vi "ALTS-2015 Delete User Account v1.0.vi"(8 "error in (no error)":errorcluster, 11 "Last User":string) -> (0 "error out":errorcluster)   [LabVIEW 2013]
panel:
  in  "Case Constant\n(See Context Help)":bool
  out "Time":string
  in  "User Name":i32(ring) items=["Administrator", "Senthil"]
  in  "Cancel":bool
  in  "Delete":bool
  # "Delete User Account"
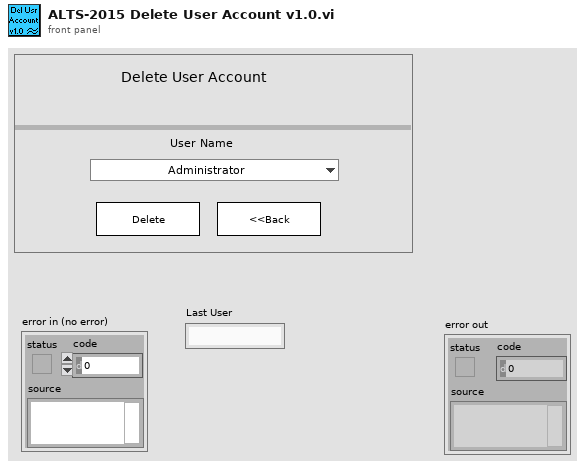
[diagram p1: front panel]
types:
  T1 = enum16{">Initialize", ">Reinitialize", ">Poll", ">Confirm Delete", ">Handle Error", ">Exit"}
  T2 = enum16{">Initialize", ">Poll", ">Confirm Delete", ">Handle Error", ">Exit"}
  T3 = typedef "ALTS-2015 User Group Enum2.ctl" = enum16{"Administrator", "Super User", "Operator"}
  T4 = cluster{"User Names":string, "Password":string, "User Rights":T3}[]
  T5 = enum16{"OK", "CANCEL", "ABORT", "RETRY", "IGNORE", "YES", "NO"}
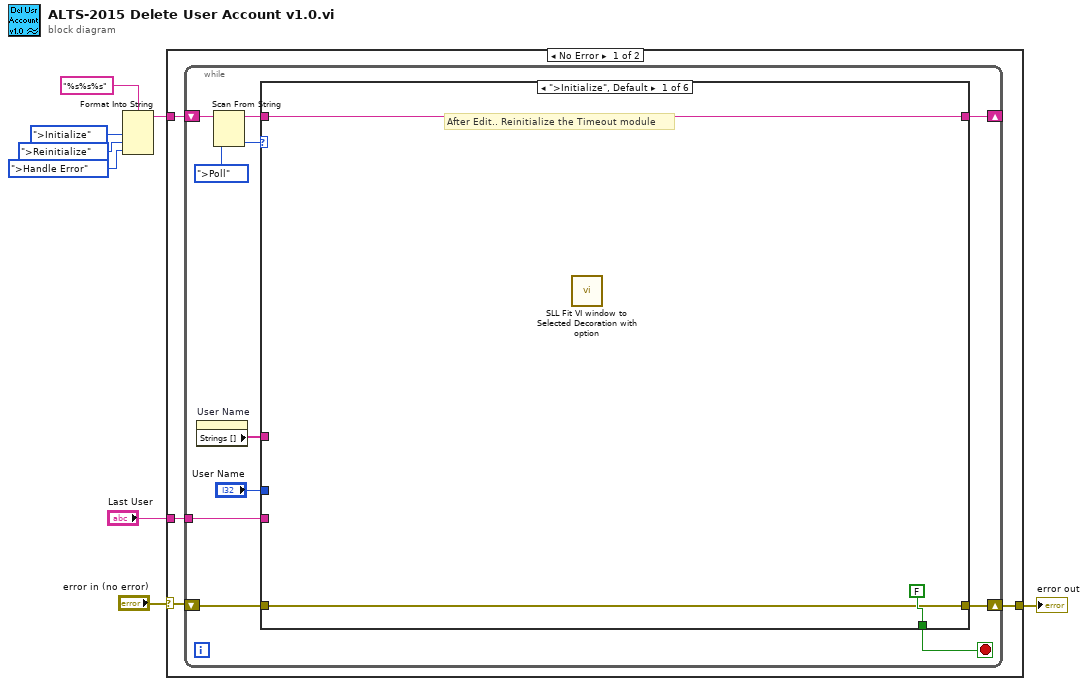
[diagram p0: block diagram]
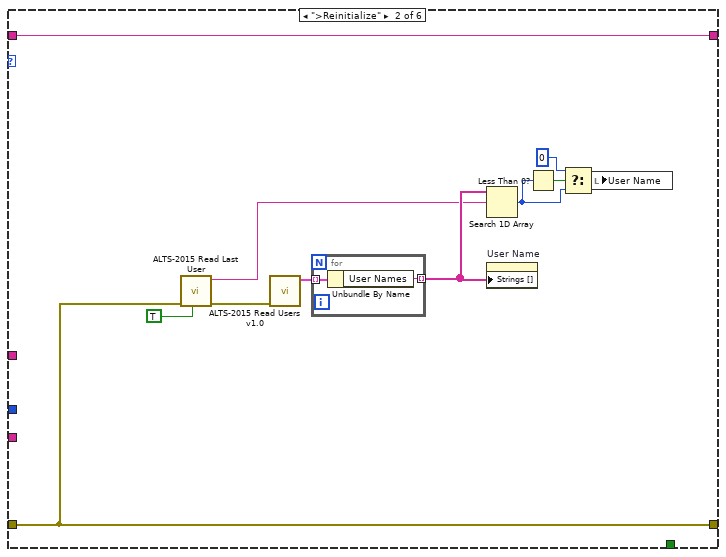
[diagram p2: hidden frame]
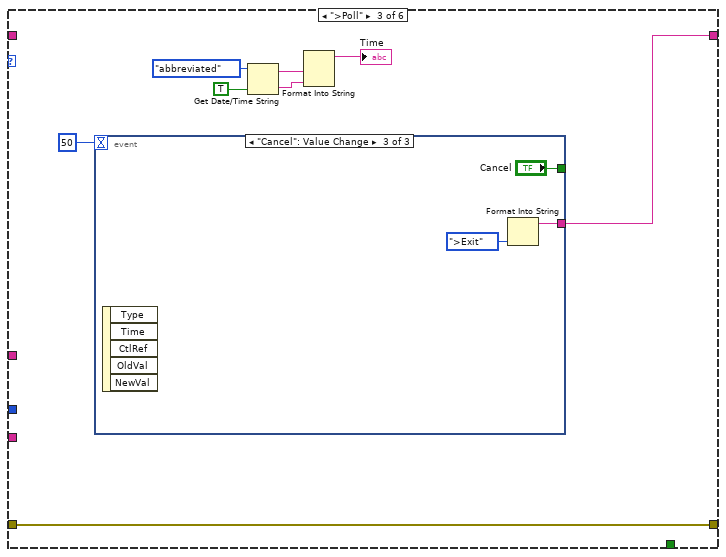
[diagram p3: hidden frame]
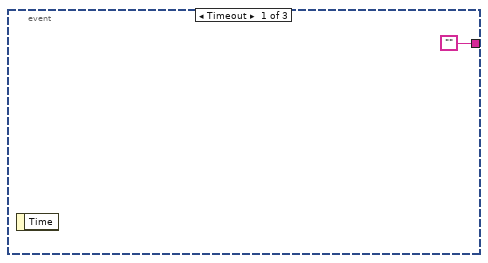
[diagram p4: hidden frame]
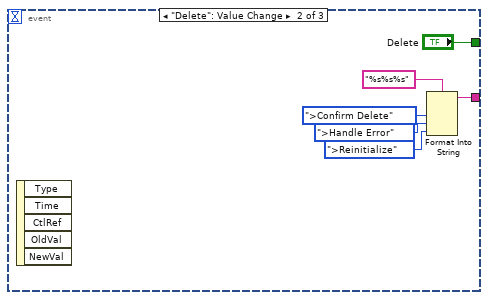
[diagram p5: hidden frame]
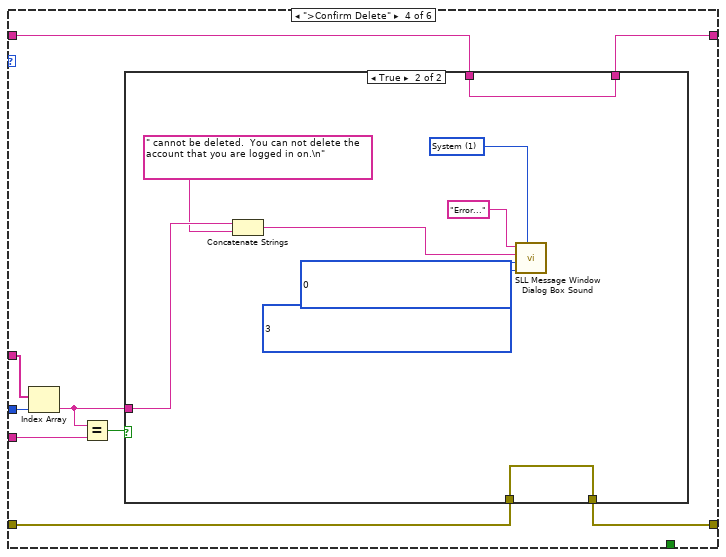
[diagram p6: hidden frame]
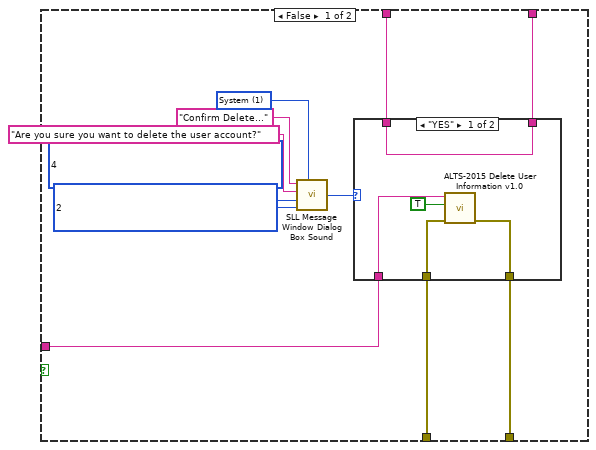
[diagram p7: hidden frame]
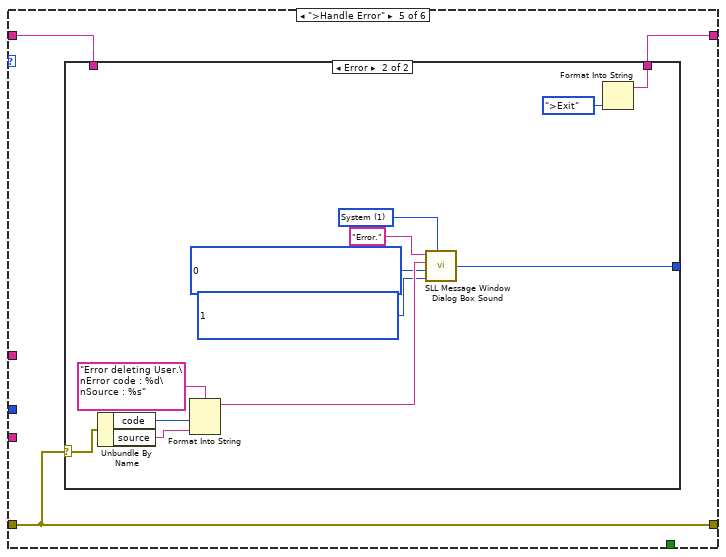
[diagram p9: hidden frame]
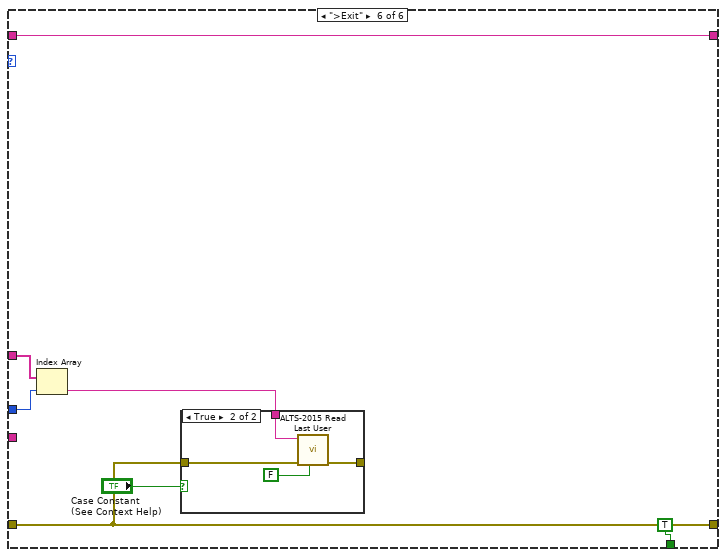
[diagram p11: hidden frame]
diagram:
  n1 = Format Into String(format string="%s%s%s", T1.">Initialize", T1.">Reinitialize", T1.">Handle Error") -> (resulting string=w5:string)  [unwired: 2 in, 1 out]
  n2 = case shown="No Error" "error in (no error)" {
    selector: "error in (no error)" -> [w12 w120]
    tunnel: [w11 w120] -> w7
    tunnel: w5 -> [w10 _]
    tunnel: "Last User" -> [w9 _]
    frame No Error {
      n3 = while {
        shift-right: [w22] -> w11
        shift-left: w12 -> [w23]
        shift-right: [w18] -> _
        shift-left: w10 -> [w21]
        tunnel: w9 -> [w13]
        stop <- w17 stop-if-true
        n4 = property on="User Name" class="Ring (strict)"() -> ("Strings []"=w14:string[])  [unwired: 2 in, 2 out]
        n5 = Scan From String(input string=w21, default 1=T1.">Poll") -> (remaining string=w19:string, output 1=w20:T1)  [unwired: 3 in, 2 out]
        n6 = case shown="\">Initialize\", Default" w20 {
          tunnel: w23 -> [w24 w27 w47 w64 w92 w108]
          tunnel: [w24 w27 w47 w63 w92 w108] -> w22
          tunnel: [w26 w37 w40 w65 w93 w114] -> w18
          tunnel: w19 -> [w26 w37 _ w66 w94 w114]
          tunnel: [FALSE _ _ _ _ TRUE] -> w17
          tunnel: "User Name" -> [_ _ _ w62 _ w111]
          tunnel: w14 -> [_ _ _ w61 _ w112]
          tunnel: w13 -> [_ _ _ w59 _ _]
          frame ">Initialize", Default {
            # "After Edit.. Reinitialize the Timeout module"
            n7 = call <userlib>:"SLL Fit VI window to Selected Decoration with option.vi"() -> ()  [unwired: 10 in, 2 out]
          }
          frame ">Reinitialize" {
            n8 = call "ALTS-2015 Read Last User.vi"("Read?"=TRUE, "error in (no error)"=w27) -> ("error out"=w28:errorcluster, "Last User"=w29:string)  [unwired: 8 in]
            n9 = call "ALTS-2015 Read Users v1.0.vi"("error in (no error)"=w28) -> ("Users"=w36:T4)  [unwired: 9 in, 1 out]
            n10 = for {
              tunnel: w36 -> [w39] mode=indexing
              tunnel: [w38] -> w35 mode=indexing
              n11 = Unbundle By Name(w39) -> ("User Names"=w38:string)
            }
            n12 = Search 1D Array(1D array=w35, element=w29) -> (index of element=w33:i32)  [unwired: 1 in]
            n13 = property on="User Name" class="Ring (strict)"("Strings []"=w35) -> ()  [unwired: 2 in, 2 out]
            n14 = Less Than 0?(x=w33) -> (x < 0?=w34:bool)
            n15 = Select(t=0, s=w34, f=w33) -> (s? t:f=w32:i32)
            n16 = local write "User Name"(w32) -> ()
          }
          frame ">Poll" {
            n17 = event shown="[2] \"Cancel\": Value Change" {
              selector: _ -> [_ _ _]
              dyn-events: _ -> [_ _ _]
              timeout: 50 -> [_ _ _]
              tunnel: ["" w53 w57] -> w40
              tunnel: [_ "Delete" "Cancel"] -> _
              event Timeout {
                n18 = event-data() -> ()  [unwired: 1 in, 1 out]
              }
              event "Delete": Value Change {
                n19 = event-data() -> ()  [unwired: 1 in, 5 out]
                n20 = Format Into String(format string="%s%s%s", T1.">Confirm Delete", T1.">Handle Error", T1.">Reinitialize") -> (resulting string=w53:string)  [unwired: 2 in, 1 out]
              }
              event "Cancel": Value Change {
                n21 = event-data() -> ()  [unwired: 1 in, 5 out]
                n22 = Format Into String(T1.">Exit") -> (resulting string=w57:string)  [unwired: 3 in, 1 out]
              }
            }
            n23 = Get Date/Time String(date format (0)=enum16{"short", "long", "abbreviated"}."abbreviated", want seconds? (F)=TRUE) -> (date string=w44:string, time string=w43:string)  [unwired: 1 in]
            n24 = Format Into String(w44, w43) -> (resulting string=→"Time":string)  [unwired: 3 in, 1 out]
          }
          frame ">Confirm Delete" {
            n25 = Index Array(array=w61, index=w62) -> (element=w60:string)
            n26 = Equal?(x=w60, y=w59) -> (x = y?=w58:bool)
            n27 = case shown="True" w58 {
              tunnel: w66 -> [w71 w91]
              tunnel: [w70 w91] -> w65
              tunnel: w64 -> [w69 w90]
              tunnel: [w68 w90] -> w63
              tunnel: w60 -> [w67 w85]
              frame False {
                w77 = 1 items=["Application", "System", "Task"] ("modality (0)")
                n28 = call <userlib>:"SLL Message Window Dialog Box Sound.vi"("Modality (0)"=w77, "Icon (0:None)"=2 ("icon (0:None)"), "Buttons (0:OK)"=4 ("buttons (0:OK)"), "Message (\"\")"="Are you sure you want to delete the user account?" ("message (\"\")"), "Window Title (\"\")"="Confirm Delete..." ("window title (\"\")")) -> ("Button Pressed"=w72:T5)  [unwired: 1 in]
                n29 = case shown="\"YES\"" w72 {
                  tunnel: w71 -> [w82 _]
                  tunnel: [w82 _] -> w70
                  tunnel: w67 -> [w78 _]
                  tunnel: w69 -> [w80 _]
                  tunnel: [w79 _] -> w68
                  frame "YES" {
                    n30 = call "ALTS-2015 Delete User Information v1.0.vi"("error in (no error)"=w80, "Add(T)/Edit(F)"=TRUE, "User Name"=w78) -> ("error out"=w79:errorcluster)  [unwired: 7 in, 1 out]
                  }
                  frame "NO", Default {
                  }
                }
              }
              frame True {
                w86 = 1 items=["Application", "System", "Task"] ("modality (0)")
                n31 = Concatenate Strings(w85, " cannot be deleted.  You can not delete the account that you are logged in on.\n") -> (w83:string)
                n32 = call <userlib>:"SLL Message Window Dialog Box Sound.vi"("Modality (0)"=w86, "Icon (0:None)"=3 ("icon (0:None)"), "Buttons (0:OK)"=0 ("buttons (0:OK)"), "Message (\"\")"=w83, "Window Title (\"\")"="Error...") -> ()  [unwired: 1 in, 1 out]
              }
            }
          }
          frame ">Handle Error" {
            n33 = case shown="Error" w92 {
              selector: w92 -> [_ w103]
              tunnel: w94 -> [w95 _]
              tunnel: [w95 w106] -> w93
              tunnel: [_ w96] -> _
              frame No Error {
              }
              frame Error {
                w104 = 1 items=["Application", "System", "Task"] ("modality (0)")
                n34 = Unbundle By Name(w103) -> ("code"=w102:i32, "source"=w101:string)
                n35 = Format Into String(format string="Error deleting User.\nError code : %d\nSource : %s", w102, w101) -> (resulting string=w99:string)  [unwired: 2 in, 1 out]
                n36 = call <userlib>:"SLL Message Window Dialog Box Sound.vi"("Modality (0)"=w104, "Icon (0:None)"=1 ("icon (0:None)"), "Buttons (0:OK)"=0 ("buttons (0:OK)"), "Message (\"\")"=w99, "Window Title (\"\")"="Error." ("window title (\"\")")) -> ("Button Pressed"=w96:T5)  [unwired: 1 in]
                n37 = Format Into String(T2.">Exit") -> (resulting string=w106:string)  [unwired: 3 in, 1 out]
              }
            }
          }
          frame ">Exit" {
            n38 = Index Array(array=w112, index=w111) -> (element=w110:string)
            n39 = case shown="True" "Case Constant\n(See Context Help)" {
              tunnel: w108 -> [w115 w119]
              tunnel: [w115 w118] -> _
              tunnel: w110 -> [_ w117]
              frame False {
              }
              frame True {
                n40 = call "ALTS-2015 Read Last User.vi"("Read?"=FALSE, "error in (no error)"=w119, "Last User"=w117) -> ("error out"=w118:errorcluster)  [unwired: 7 in, 1 out]
              }
            }
          }
        }
      }
    }
    frame Error {
    }
  }
  "error out" <- w7
